vi "VMI_IO_date_file.vi"(3 "Error In":errorcluster, 4 "File date in":string="120416aa", 5 "File Task":u16(ring) items=["Read", "Write"]) -> (0 "Error Out":errorcluster, 2 "File date out":string)   [LabVIEW 2019]
panel:
  out "appended path":path
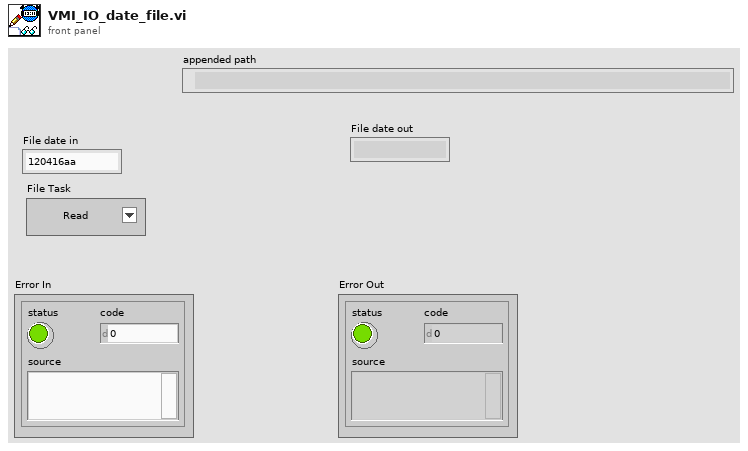
[diagram p1: front panel]
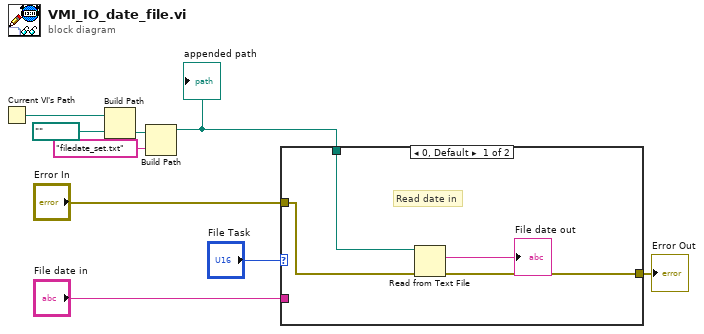
[diagram p0: block diagram]
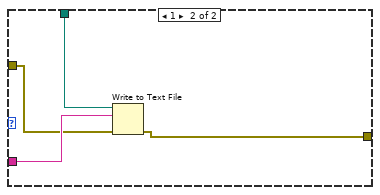
[diagram p2: hidden frame]
diagram:
  n1 = Current VI's Path() -> (path=w7:path)
  n2 = Build Path(base path=w7, name or relative path=path "..") -> (appended path=w6:path)
  n3 = Build Path(base path=w6, name or relative path="filedate_set.txt") -> (appended path=w4:path)
  "appended path" <- w4
  n4 = case shown="0, Default" "File Task" {
    tunnel: w4 -> [w13 w17]
    tunnel: "File date in" -> [_ w16]
    tunnel: "Error In" -> [w12 w15]
    tunnel: [w11 w14] -> w1
    frame 0, Default {
      # "Read date in"
      n5 = Read from Text File(file (use dialog)=w13, error in=w12) -> (text=→"File date out":string, error out=w11:errorcluster)  [unwired: 2 in, 2 out]
    }
    frame 1 {
      n6 = Write to Text File(file (use dialog)=w17, text=w16, error in=w15) -> (error out=w14:errorcluster)  [unwired: 1 in, 2 out]
    }
  }
  "Error Out" <- w1
